vi "AIT 1553 - Parse Tree Parameters.vi"(6 "Access Type":T1=enum."Write", 7 "Bus Section":T2, 8 "error in":errorcluster, 11 "Item Ref in":T6 format="%.0x") -> (0 "error out":errorcluster, 2 "Parameter References":T6[](array[typedef]) format="%.0x", 3 "Item Ref out":T6 format="%.0x", 4 "Parameter Driver Data":T3 {"First Word" min=8 max=31; "Num Bits" min=1 max=32; "Start Bit" min=8 max=31})   [LabVIEW 2013, in "AIT 1553 Custom Device.lvlib"]
uses:
  AIT 1553 Custom Device.lvlib
  <vilib>/NI Veristand/Custom Device API/Custom Device Item Ref.ctl
  RT Controls/AIT 1553 - Driver Data.ctl
  Controls and Global/Start Bit.ctl
  Controls and Global/Number of Bits.ctl
  RT Controls/AIT 1553 - Bus Section.ctl
  <vilib>/NI Veristand/Custom Device API/Data Access Type.ctl
  <vilib>/NI Veristand/Custom Device Tools/Custom Device Utility Library/RT Debug String Color Spec.ctl
  Controls and Global/Global.vi
  <vilib>/NI Veristand/Custom Device Tools/Custom Device Utility Library/NI VeriStand - Search for All Items by GUID.vi
  <vilib>/NI Veristand/Custom Device Tools/Custom Device Utility Library/NI VeriStand - Search for Item by GUID.vi
  <vilib>/NI Veristand/Custom Device API/Get Item Property (Double).vi
  <vilib>/NI Veristand/Custom Device API/Get Item Property (Boolean).vi
  <vilib>/NI Veristand/Custom Device API/Get Item Property (I32).vi
  <vilib>/NI Veristand/Custom Device API/Custom Device API.lvlib
  <vilib>/NI Veristand/Custom Device Tools/Custom Device Utility Library/Custom Device Utility Library.lvlib
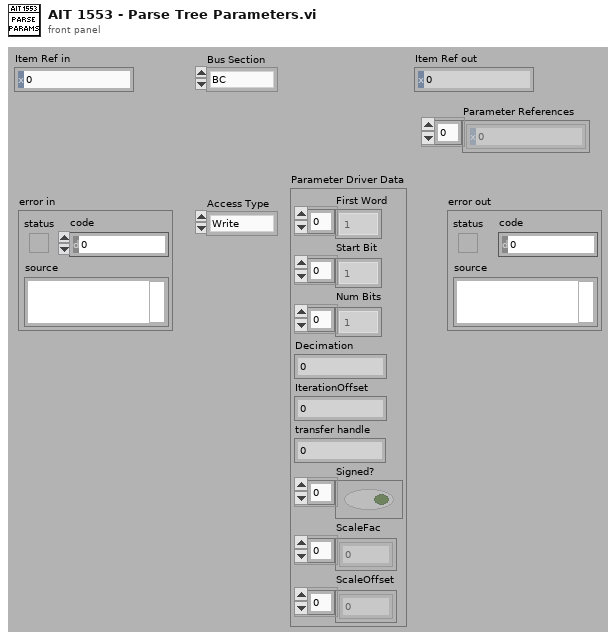
[diagram p1: front panel]
types:
  T1 = typedef "Custom Device API.lvlib/Data Access Type.ctl" = enum16{"Read", "Write"}
  T2 = typedef "AIT 1553 Custom Device.lvlib/AIT 1553 - Bus Section.ctl" = enum16{"BC", "BM", "RT"}
  T3 = typedef "AIT 1553 Custom Device.lvlib/AIT 1553 - Driver Data.ctl" = cluster{"First Word":T4[], "Start Bit":T4[], "Num Bits":T5[], "Decimation":i32, "IterationOffset":i32, "transfer handle":u32, "Signed?":bool[], "ScaleFac":dbl[], "ScaleOffset":dbl[]}
  T4 = typedef "AIT 1553 Custom Device.lvlib/Start Bit.ctl" = i32
  T5 = typedef "AIT 1553 Custom Device.lvlib/Number of Bits.ctl" = i32
  T6 = typedef "Custom Device API.lvlib/Custom Device Item Ref.ctl" = u64
  T7 = typedef "Custom Device Utility Library.lvlib/RT Debug String Color Spec.ctl" = u16
  T8 = typedef "Custom Device API.lvlib/Custom Device Item Info.ctl" = cluster{"Name":string, "Is Channel":bool, "GUID":string, "Is Waveform":bool}
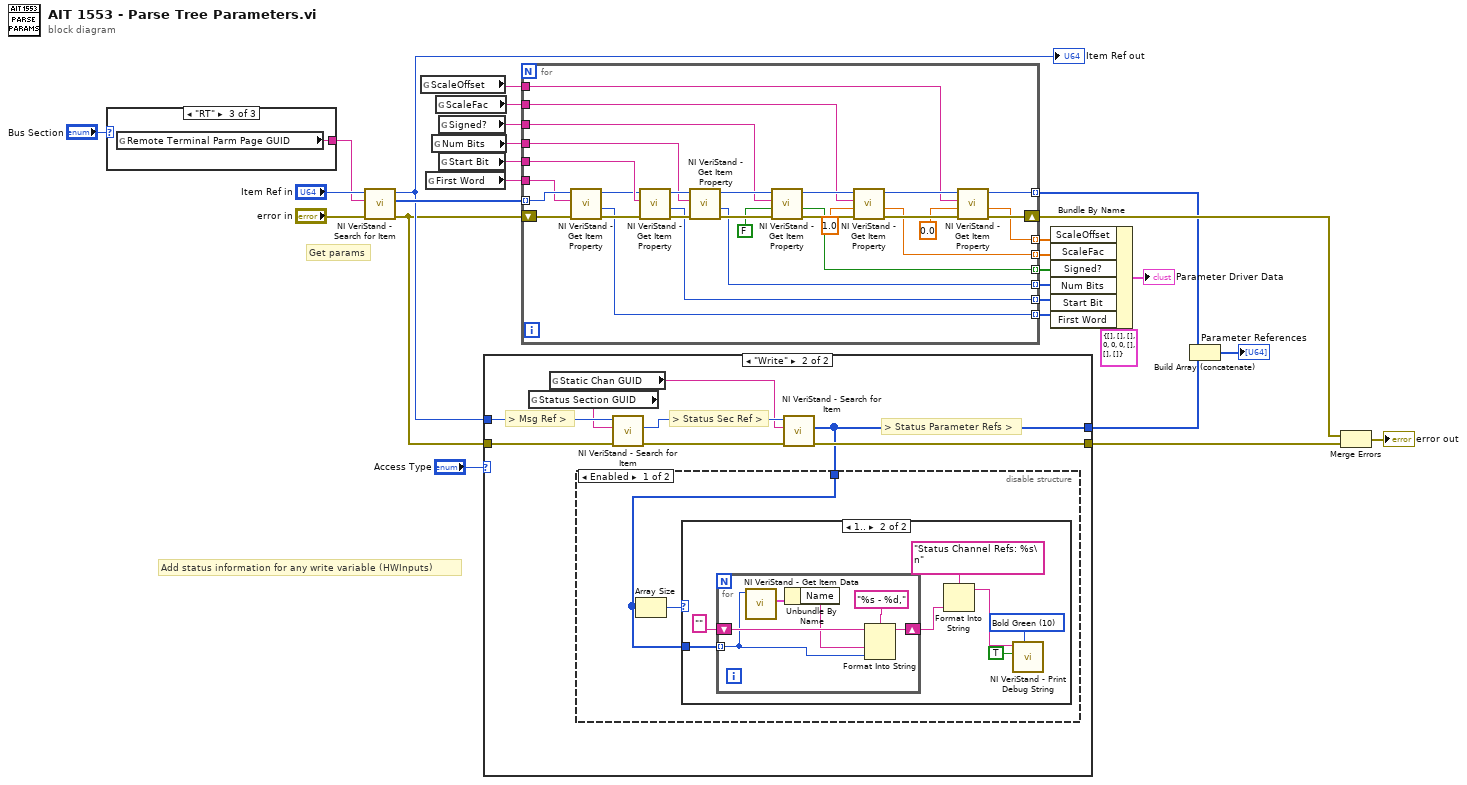
[diagram p0: block diagram]
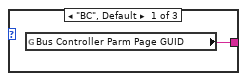
[diagram p5: hidden frame]
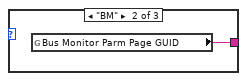
[diagram p6: hidden frame]
diagram:
  # "Add status information for any write variable (HWInputs)"
  # "Get params"
  n1 = case shown="\"RT\"" "Bus Section" {
    tunnel: [w29 w30 w31] -> w10
    frame "BC", Default {
      n2 = global read "Global.vi" "Bus Controller Parm Page GUID"() -> (w29:string)
    }
    frame "BM" {
      n3 = global read "Global.vi" "Bus Monitor Parm Page GUID"() -> (w30:string)
    }
    frame "RT" {
      n4 = global read "Global.vi" "Remote Terminal Parm Page GUID"() -> (w31:string)
    }
  }
  n5 = call-poly <vilib>:"NI VeriStand - Search for Item.vi"("error in"="error in", "Item GUID"=w10, "Section Ref in"="Item Ref in") -> ("error out"=w8:errorcluster, "Item Refs"=w24:T6[], "Section Ref out"=w9:T6)  [unwired: 5 in, 1 out]
  "Item Ref out" <- w9
  n6 = global read "Global.vi" "ScaleOffset"() -> (w21:string)
  n7 = global read "Global.vi" "First Word"() -> (w18:string)
  n8 = global read "Global.vi" "Num Bits"() -> (w28:string)
  n9 = global read "Global.vi" "ScaleFac"() -> (w22:string)
  n10 = global read "Global.vi" "Signed?"() -> (w23:string)
  n11 = global read "Global.vi" "Start Bit"() -> (w27:string)
  n12 = case shown="\"Write\"" "Access Type" {
    tunnel: w9 -> [_ w40]
    tunnel: w8 -> [w32 w39]
    tunnel: [w32 w34] -> w6
    tunnel: [_ w33] -> w3
    frame "Read", Default {
    }
    frame "Write" {
      # "> Status Parameter Refs >"
      # "> Status Sec Ref >"
      # "> Msg Ref >"
      n13 = global read "Global.vi" "Status Section GUID"() -> (w38:string)
      n14 = global read "Global.vi" "Static Chan GUID"() -> (w35:string)
      n15 = call-poly <vilib>:"NI VeriStand - Search for Item.vi"("error in"=w39, "Item GUID"=w38, "Section Ref in"=w40) -> ("error out"=w37:errorcluster, "Item Ref"=w36:T6)  [unwired: 5 in, 2 out]
      n16 = call-poly <vilib>:"NI VeriStand - Search for Item.vi"("error in"=w37, "Item GUID"=w35, "Section Ref in"=w36) -> ("error out"=w34:errorcluster, "Item Refs"=w33:T6[])  [unwired: 5 in, 2 out]
      n17 = disable-structure shown="Enabled" {
        disable-tunnel: w33 -> [w41 _]
        frame Enabled {
          n18 = Array Size(array=w41) -> (size(s)=w42:i32)
          n19 = case shown="1.." w42 {
            tunnel: w41 -> [_ w48]
            frame 0, Default {
            }
            frame 1.. {
              w44 = T7 10 items=["Plain White"=7, "Bold White"=15, "Bold Blue"=9, "Bold Green"=10, "Bold Red"=12] ("Attribute")
              n20 = for {
                tunnel: w48 -> [w52] mode=indexing
                shift-right: [w53] -> w46
                shift-left: "" ("format string") -> [w54]
                n21 = call <vilib>:"NI VeriStand - Get Item Data.vi"("Item Ref in"=w52) -> ("Item Info"=w51:T8)  [unwired: 7 in, 3 out]
                n22 = Unbundle By Name(w51) -> ("Name"=w50:string)
                n23 = Format Into String(format string="%s - %d,", initial string=w54, w50, w52) -> (resulting string=w53:string)  [unwired: 1 in, 1 out]
              }
              n24 = Format Into String(format string="Status Channel Refs: %s\n", w46) -> (resulting string=w45:string)  [unwired: 2 in, 1 out]
              n25 = call <vilib>:"NI VeriStand - Print Debug String.vi"("Attribute"=w44, "Add to log file? (T)"=TRUE, "Message"=w45) -> ()  [unwired: 8 in, 1 out]
            }
          }
        }
        frame Disabled {
        }
      }
    }
  }
  n26 = for {
    shift-right: [w75] -> w7
    shift-left: w8 -> [w68]
    tunnel: w24 -> [w67] mode=indexing
    tunnel: w27 -> [w82]
    tunnel: w28 -> [w81]
    tunnel: [w80] -> w16 mode=indexing
    tunnel: [w76] -> w4 mode=indexing
    tunnel: w23 -> [w71]
    tunnel: w22 -> [w62]
    tunnel: w21 -> [w63]
    tunnel: w18 -> [w66]
    tunnel: [w61] -> w17 mode=indexing
    tunnel: [w60] -> w15 mode=indexing
    tunnel: [w59] -> w14 mode=indexing
    tunnel: [w57] -> w13 mode=indexing
    tunnel: [w56] -> w12 mode=indexing
    n27 = call-poly <vilib>:"NI VeriStand - Get Item Property.vi"("error in (no error)"=w68, "Property Name"=w66, "Item Ref in"=w67) -> ("error out"=w64:errorcluster, "Value"=w61:i32, "Item Ref out"=w65:T6)  [unwired: 5 in, 1 out]
    n28 = call-poly <vilib>:"NI VeriStand - Get Item Property.vi"("error in (no error)"=w64, "Property Name"=w82, "Item Ref in"=w65) -> ("error out"=w84:errorcluster, "Value"=w80:i32, "Item Ref out"=w83:T6)  [unwired: 5 in, 1 out]
    n29 = call-poly <vilib>:"NI VeriStand - Get Item Property.vi"("error in (no error)"=w84, "Property Name"=w81, "Item Ref in"=w83) -> ("error out"=w72:errorcluster, "Value"=w60:i32, "Item Ref out"=w79:T6)  [unwired: 5 in, 1 out]
    n30 = call-poly <vilib>:"NI VeriStand - Get Item Property.vi"("error in (no error)"=w72, "Default Value"=FALSE, "Property Name"=w71, "Item Ref in"=w79) -> ("error out"=w73:errorcluster, "Value"=w59:bool, "Item Ref out"=w78:T6)  [unwired: 4 in, 1 out]
    n31 = call-poly <vilib>:"NI VeriStand - Get Item Property.vi"("error in (no error)"=w73, "Default Value"=1.0, "Property Name"=w62, "Item Ref in"=w78) -> ("error out"=w74:errorcluster, "Value"=w57:dbl, "Item Ref out"=w77:T6)  [unwired: 4 in, 1 out]
    n32 = call-poly <vilib>:"NI VeriStand - Get Item Property.vi"("error in (no error)"=w74, "Default Value"=0.0, "Property Name"=w63, "Item Ref in"=w77) -> ("error out"=w75:errorcluster, "Value"=w56:dbl, "Item Ref out"=w76:T6)  [unwired: 4 in, 1 out]
  }
  n33 = Bundle By Name(cluster=T3 {"First Word"=[], "Start Bit"=[], "Num Bits"=[], "Decimation"=0, "IterationOffset"=0, "transfer handle"=0, "Signed?"=[], "ScaleFac"=[], "ScaleOffset"=[]} ("Parameter Driver Data"), "ScaleOffset"=w12, "ScaleFac"=w13, "Signed?"=w14, "Num Bits"=w15, "Start Bit"=w16, "First Word"=w17) -> (→"Parameter Driver Data":T3)
  n34 = Build Array (concatenate)(w4, w3) -> (→"Parameter References":T6[])
  n35 = Merge Errors(w7, w6) -> (→"error out":errorcluster)
